vi "Barcode Checker.vi"() -> ()   [LabVIEW 2015]
panel:
  out "Barcodes (Barcode Reader 1)":T1(array[cluster]) {"Confidence Level" format="%.2f"; "Barcode Type" items=["Reserved", "Codabar", "Code 39", "Code 93", "Code 128", "EAN 8", "EAN 13", "Interleaved 2 of 5", "MSI", "UPCA", "Pharmacode", "RSS Limited"]; "Bounding Box"."y" format="%.2f"; "Bounding Box"."x" format="%.2f"}
  out "fps":dbl(knob) scale=0.0..45.0
  out "Frame Rate":dbl
  in  "Stop (F)":bool
  out "Image Out":T2(plugin-control)
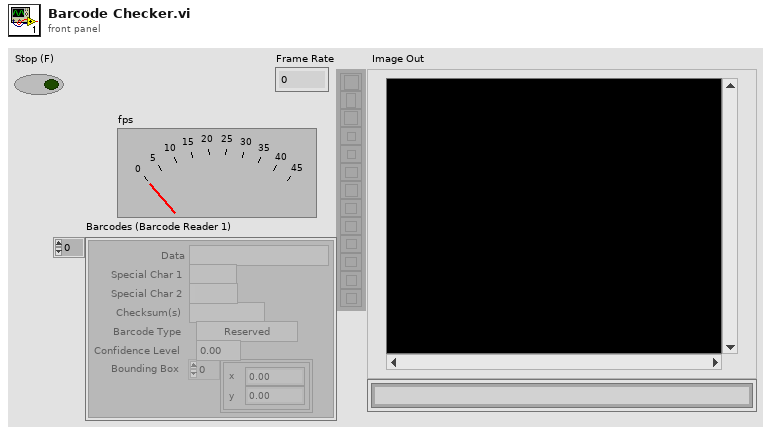
[diagram p1: front panel]
types:
  T1 = cluster{"Data":string, "Special Char 1":string, "Special Char 2":string, "Checksum(s)":string, "Barcode Type":u32, "Confidence Level":sgl, "Bounding Box":cluster{"x":sgl, "y":sgl}[]}[]
  T2 = typedef "IMAQ Image.ctl" = refnum<image>
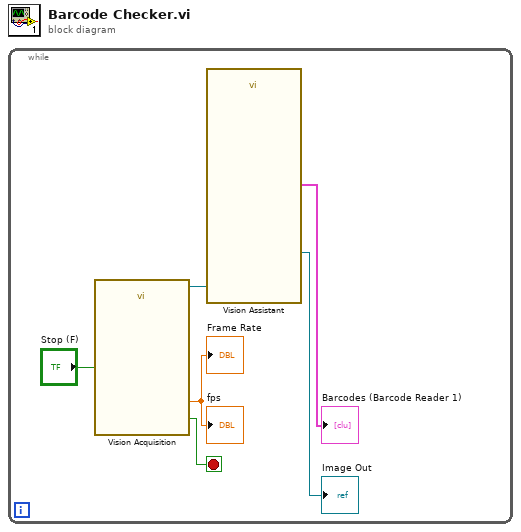
[diagram p0: block diagram]
diagram:
  n1 = while {
    stop <- w5 stop-if-true
    n2 = call "Vision Acquisition"("Stop (F)"="Stop (F)") -> ("Image Out"=w3:T2, "Frame Rate"=→"Frame Rate" →"fps":dbl, "Stopped"=w5:bool)  [unwired: 22 in, 2 out]
    n3 = call "Vision Assistant"("Image In"=w3) -> ("Image Out"=→"Image Out":T2, "Barcodes (Barcode Reader 1)"=→"Barcodes (Barcode Reader 1)":T1)  [unwired: 21 in, 4 out]
  }
